vi "Rinocloud_project_selector.vi"() -> (3 "Status":T1(ring))   [LabVIEW 2013]
panel:
  in  "Cancel Button":bool
  in  "OK Button":bool
  in  "Project":string(combo)
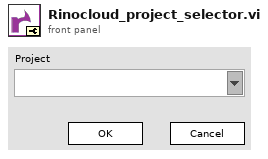
[diagram p1: front panel]
types:
  T1 = enum16{"Boot", "Initialize", "Wait for event", "Refresh", "Metadata to tree", "Stop"}
  T2 = enum32{"Invalid", "Standard", "Closed", "Hidden", "Minimized", "Maximized"}
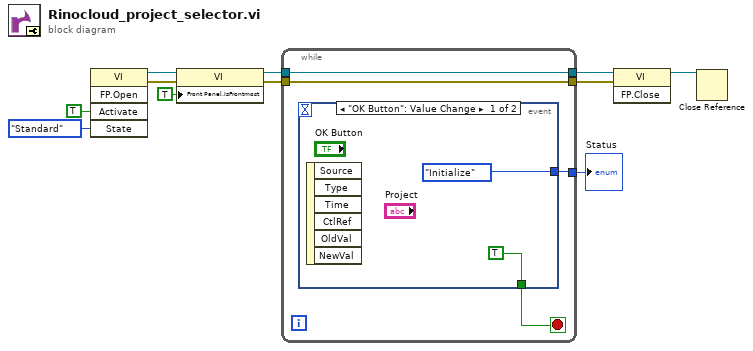
[diagram p0: block diagram]
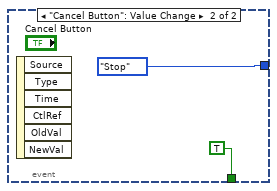
[diagram p2: hidden frame]
diagram:
  n1 = invoke class="VI" method="FP.Open"("Activate"=TRUE ("Activate?"), "State"=T2."Standard") -> (reference out=w8:refnum<vi>, error out=w4:errorcluster)  [unwired: 3 in, 3 out]
  n2 = property class="VI"(reference=w8, error in=w4, "Front Panel.IsFrontmost"=TRUE ("Front Panel Window:Is Frontmost")) -> (reference out=w7:refnum<vi>, error out=w3:errorcluster)
  n3 = while {
    tunnel: [w15] -> w9
    tunnel: w3 -> [w15]
    tunnel: [w13] -> w2
    tunnel: [w14] -> w6
    tunnel: w7 -> [w14]
    stop <- w12 stop-if-true
    n4 = event shown="[0] \"OK Button\": Value Change" {
      selector: _ -> [_ _]
      dyn-events: _ -> [_ _]
      timeout: _ -> [_ _]
      tunnel: [T1."Initialize" T1."Stop"] -> w13
      tunnel: [TRUE TRUE] -> w12
      event "OK Button": Value Change {
        n5 = event-data() -> ()  [unwired: 1 in, 6 out]
      }
      event "Cancel Button": Value Change {
        n6 = event-data() -> ()  [unwired: 1 in, 6 out]
      }
    }
  }
  "Status" <- w2
  n7 = invoke class="VI" method="FP.Close"(reference=w6, error in=w9) -> (reference out=w1:refnum<vi>)  [unwired: 1 in, 2 out]
  n8 = Close Reference(reference=w1) -> ()  [unwired: 1 in, 1 out]
